vi "MoveHatchIntake.vi"() -> ()   [LabVIEW 2018]
uses:
  Framework/Robot Global Data.vi
panel:
  in  "Collapsed":bool
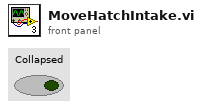
[diagram p1: front panel]
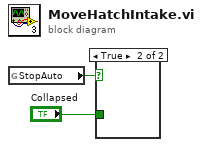
[diagram p0: block diagram]
diagram:
  n1 = global read "Robot Global Data.vi" "StopAuto"() -> (w1:bool)
  n2 = case shown="True" w1 {
    tunnel: "Collapsed" -> [_ _]
    frame False {
    }
    frame True {
    }
  }
